vi "SRV_Is Greater Than Zero.vi"(7 "Numeric (DBL)":dbl) -> (8 "Greater Than Zero":bool)   [LabVIEW 2014]
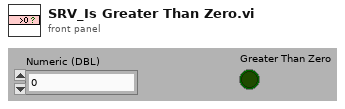
[diagram p1: front panel]
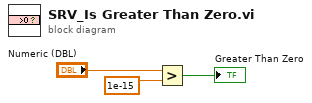
[diagram p0: block diagram]
diagram:
  n1 = Greater?(x="Numeric (DBL)", y=1e-15 ("upper limit")) -> (0:→"Greater Than Zero":bool)
